vi "XYMotion.vi"   [LabVIEW 2020]
uses:
  Aerotech.lvlib
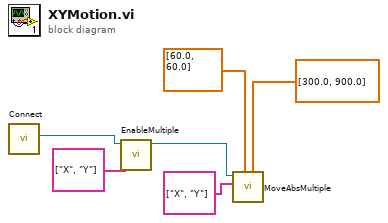
[diagram p0: block diagram]
diagram:
  n1 = call "Connect.vi"() -> ("controller"=w5:refnum<k24>)  [unwired: 10 in, 1 out]
  n2 = call "EnableMultiple.vi"("axis names"=string[] ["X", "Y"], "controller in"=w5) -> ("controller out"=w4:refnum<k24>)  [unwired: 8 in, 1 out]
  n3 = call "MoveAbsMultiple.vi"("positions"=dbl[] [300.0, 900.0], "speeds"=dbl[] [60.0, 60.0], "axis names"=string[] ["X", "Y"], "controller in"=w4) -> ()  [unwired: 6 in, 2 out]
